vi "SaveFileData.vi"(8 "error in (no error)":errorcluster, 10 "NameFile":string, 11 "ClassDataTree in":refnum<class "ClassDataTree.lvclass">) -> (0 "error out":errorcluster, 3 "ClassDataTree out":refnum<class "ClassDataTree.lvclass">)   [LabVIEW 2016, in "ClassDataTree.lvclass"]
uses:
  ClassDataTree.lvclass
  ClassDataTree.lvclass/ClassDataTree.ctl
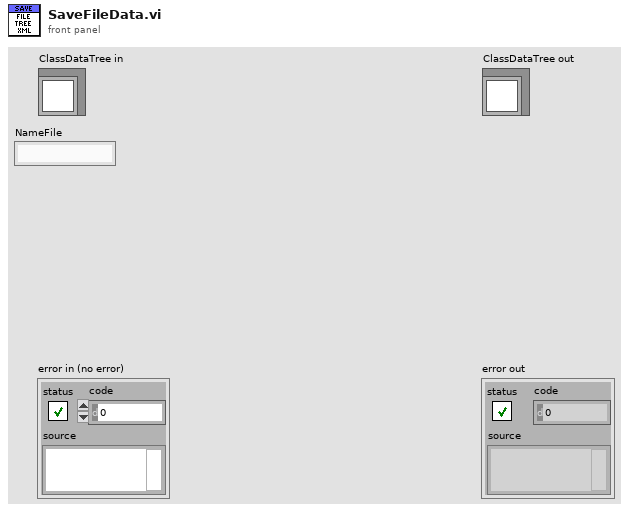
[diagram p1: front panel]
types:
  T1 = cluster{"Get Parent":string, "Active Item Tag":string, "Cell String":string, "Indent Level":i32}[]
  T2 = cluster{"Get Parent":string, "Active Item Tag":string, "Cell String":string, "Indent Level":i32}
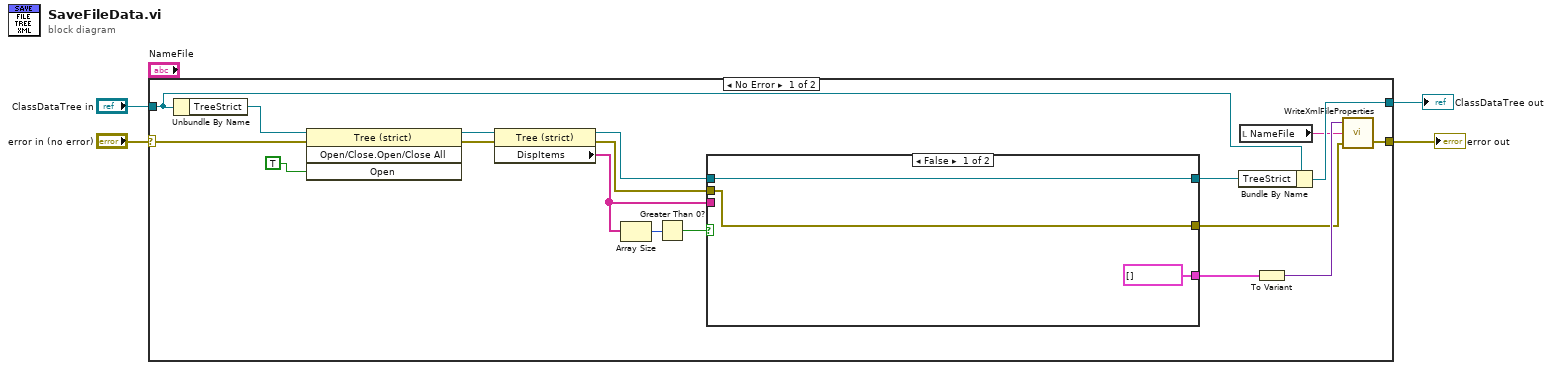
[diagram p0: block diagram]
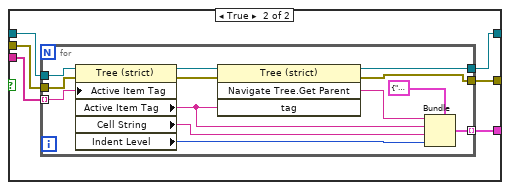
[diagram p2: hidden frame]
diagram:
  n1 = case shown="No Error" "error in (no error)" {
    selector: "error in (no error)" -> [w12 w46]
    tunnel: [w19 w46] -> w3
    tunnel: [w14 w45] -> w1
    tunnel: "ClassDataTree in" -> [w16 w45]
    frame No Error {
      n2 = Unbundle By Name(w16) -> ("TreeStrict"=w9:refnum<vi>)
      n3 = invoke class="Tree (strict)" method="Open/Close.Open/Close All"(reference=w9, error in=w12, "Open"=TRUE ("Open?")) -> (reference out=w13:refnum<vi>, error out=w10:errorcluster)  [unwired: 1 in, 2 out]
      n4 = property class="Tree (strict)"(reference=w13, error in=w10) -> (reference out=w22:refnum<vi>, error out=w18:errorcluster, "DispItems"=w7:string[])
      n5 = Array Size(array=w7) -> (size(s)=w6:i32)
      n6 = Greater Than 0?(x=w6) -> (x > 0?=w5:bool)
      n7 = case shown="False" w5 {
        tunnel: w7 -> [_ w31]
        tunnel: w22 -> [w25 w30]
        tunnel: [T1 [] w29] -> w21
        tunnel: w18 -> [w24 w28]
        tunnel: [w24 w27] -> w17
        tunnel: [w25 w26] -> w15
        frame False {
        }
        frame True {
          n8 = for {
            tunnel: w31 -> [w41] mode=indexing
            tunnel: w30 -> [w44]
            tunnel: [w43] -> w29 mode=indexing
            tunnel: w28 -> [w42]
            tunnel: [w32] -> w27
            tunnel: [w33] -> w26
            n9 = property class="Tree (strict)"(reference=w44, error in=w42, "Active Item Tag"=w41) -> (reference out=w40:refnum<vi>, error out=w39:errorcluster, "Active Item Tag"=w37:string, "Cell String"=w36:string, "Indent Level"=w35:i32)
            n10 = invoke class="Tree (strict)" method="Navigate Tree.Get Parent"(reference=w40, error in=w39, "tag"=w37) -> (reference out=w33:refnum<vi>, error out=w32:errorcluster, "Navigate Tree:Get Parent"=w38:string)  [unwired: 1 in, 1 out]
            n11 = Bundle(cluster=T2 {"Get Parent"="", "Active Item Tag"="", "Cell String"="", "Indent Level"=0}, "Get Parent"=w38, "Active Item Tag"=w37, "Cell String"=w36, "Indent Level"=w35) -> (w43:T2)
          }
        }
      }
      n12 = Bundle By Name(cluster=w16, "TreeStrict"=w15) -> (w14:refnum<class "ClassDataTree.lvclass">)
      n13 = local read "NameFile"() -> (w8:string)
      n14 = To Variant(anything=w21) -> (Variant=w20:variant)
      n15 = call "WriteXmlFileProperties.vi"("error in"=w17, "NameFileAndType"=w8, "Parameters"=w20) -> ("error out"=w19:errorcluster)  [unwired: 1 out]
    }
    frame Error {
    }
  }
  "error out" <- w3
  "ClassDataTree out" <- w1
